vi "example_tinygo_sht31_monitor.vi"() -> ()   [LabVIEW 2020]
uses:
  <vilib>/Instr/_visa.llb/VISA Configure Serial Port (Instr).vi
  <vilib>/ptbypt/NI_PtbyPt.lvlib
panel:
  out "TimeStamp":timestamp
  out "dT (ms)":u32
  out "Error Count":u32
  out "Waveform Chart":cluster{dbl, dbl}(graph)
  in  "Brn Clear":bool
  in  "Btn Send":bool
  in  "cmd string":string
  out "rcvdata counter":i32
  out "rcvdata string":string
  in  "que type":cluster{"event":string, "param":variant}
  out "read buffer":string
  in  "Btn stop":bool
  in  "VISA resource name":refnum<visa-resource-name>
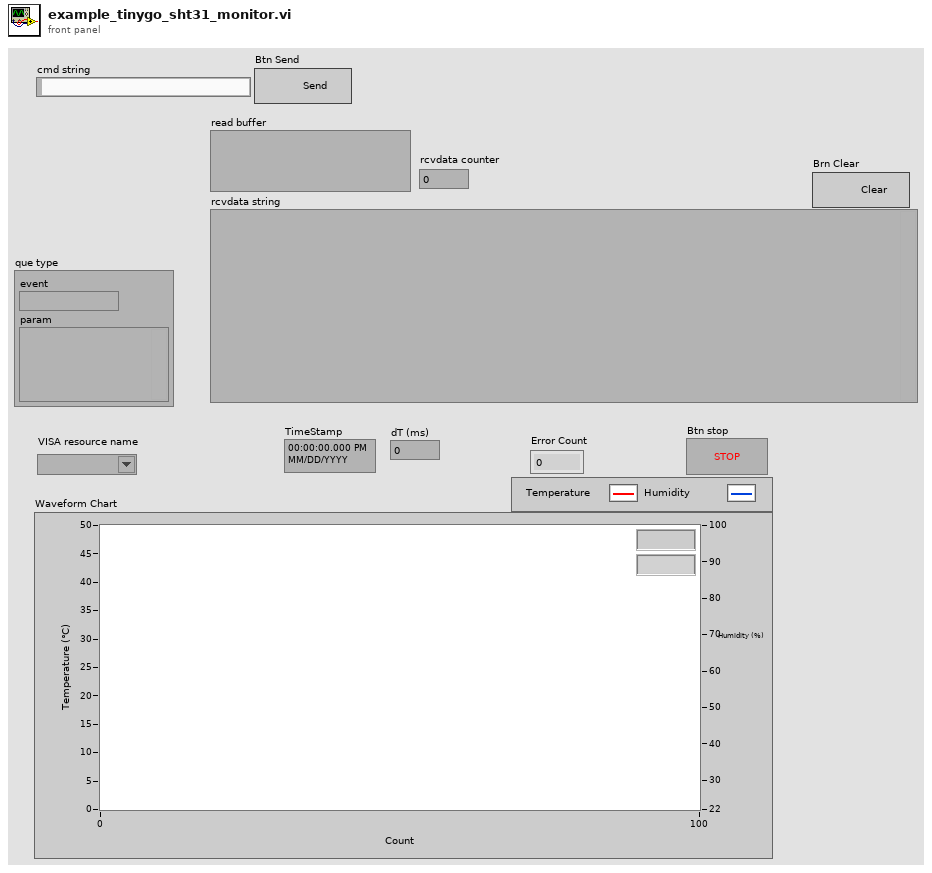
[diagram p1: front panel]
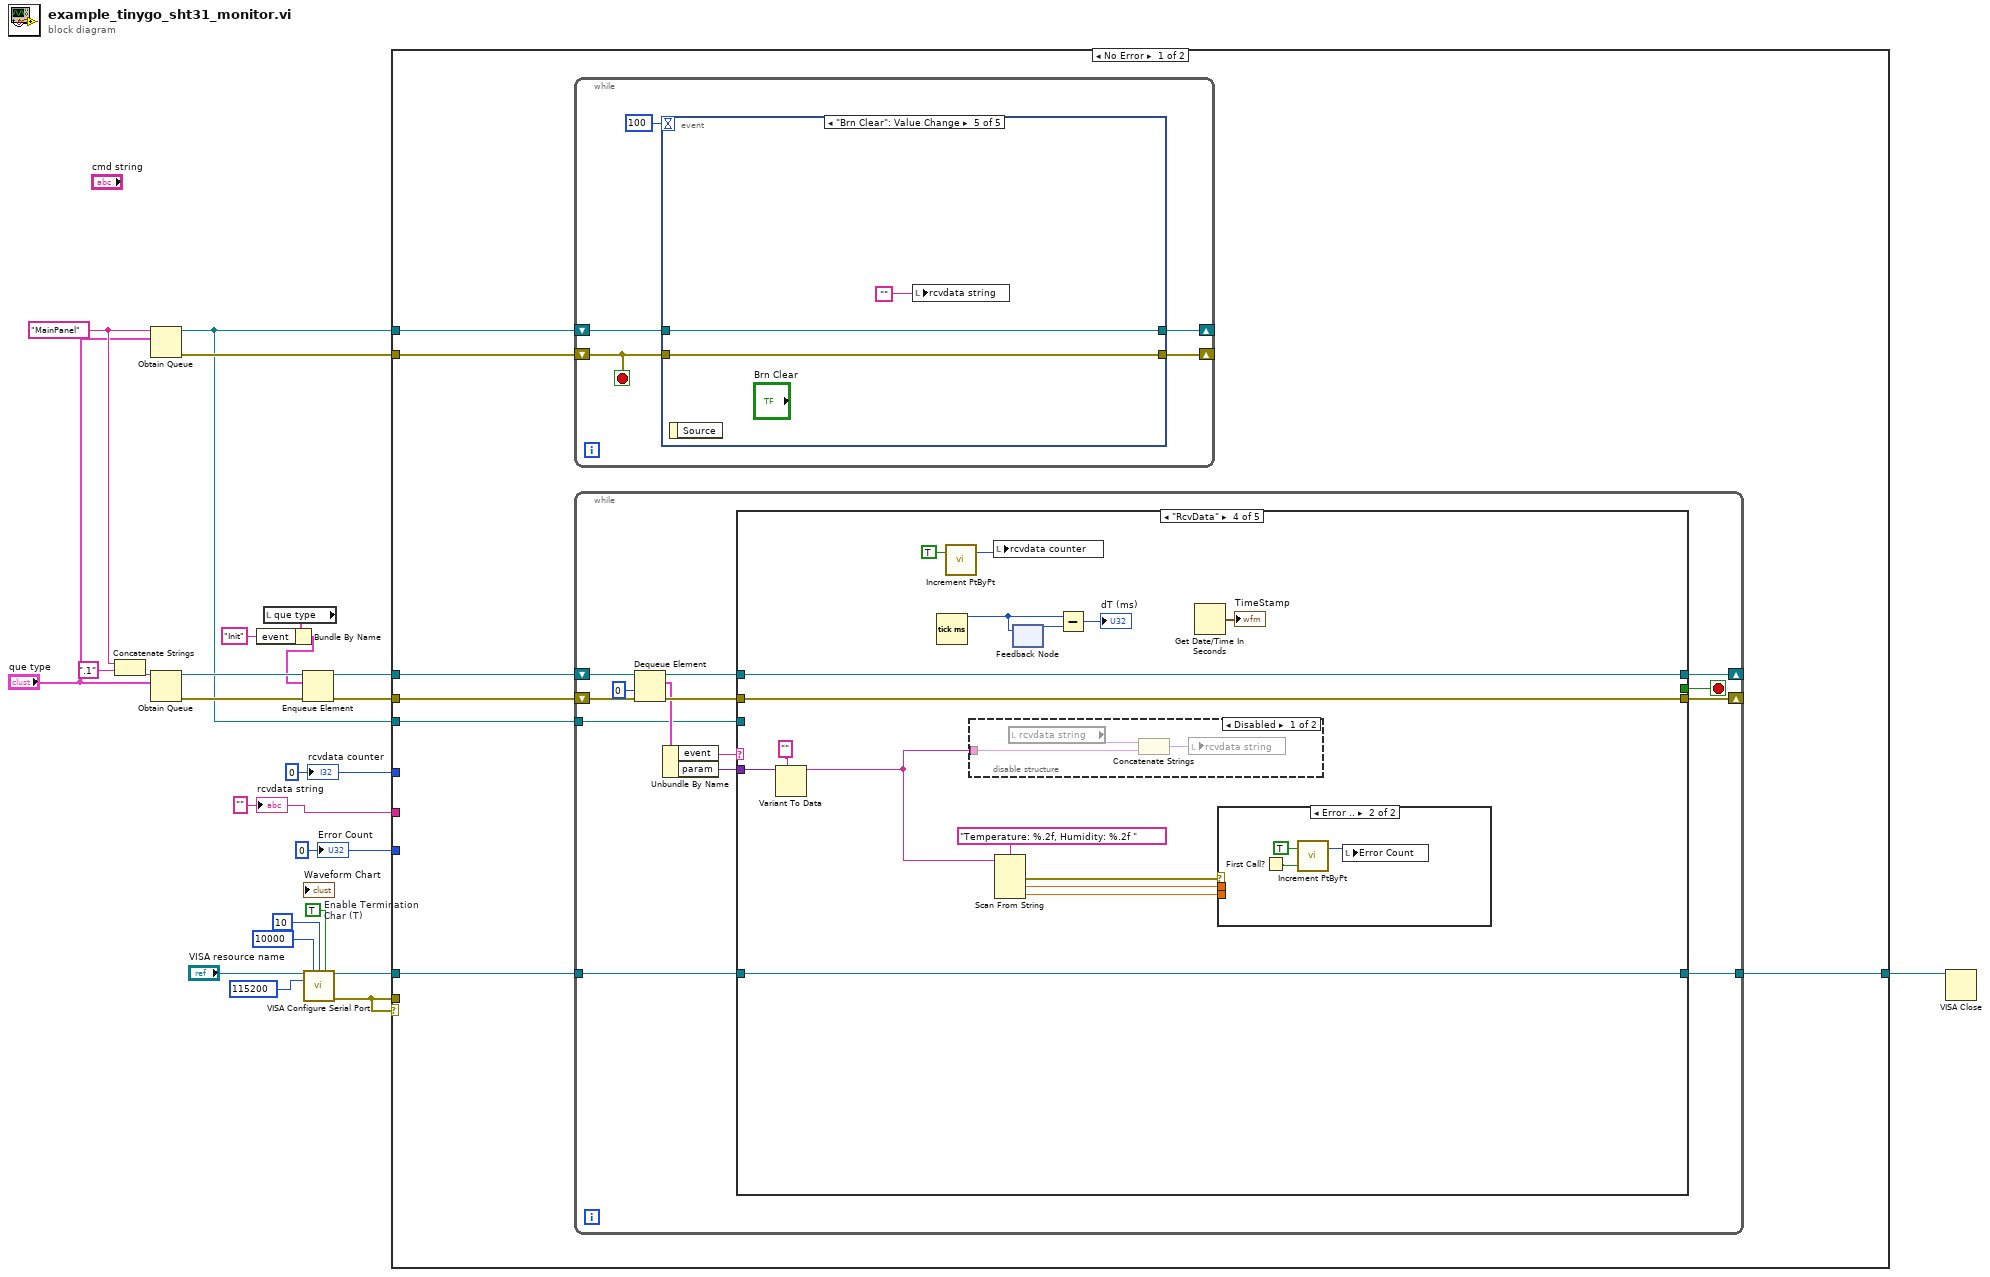
[diagram p0: block diagram]
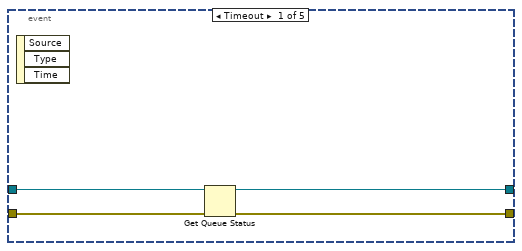
[diagram p2: hidden frame]
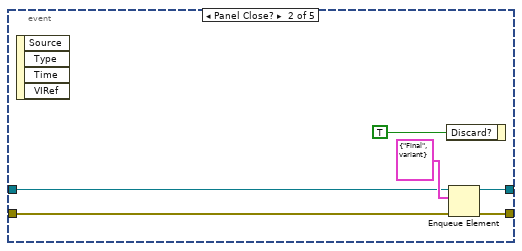
[diagram p3: hidden frame]
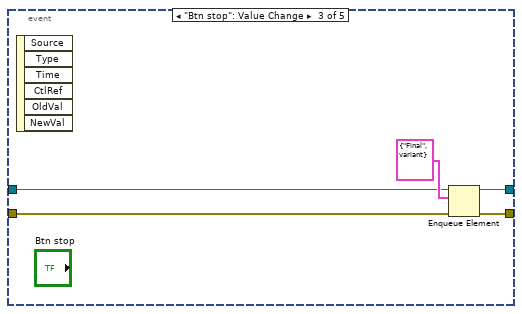
[diagram p4: hidden frame]
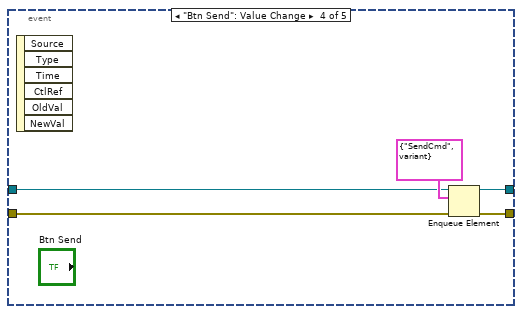
[diagram p5: hidden frame]
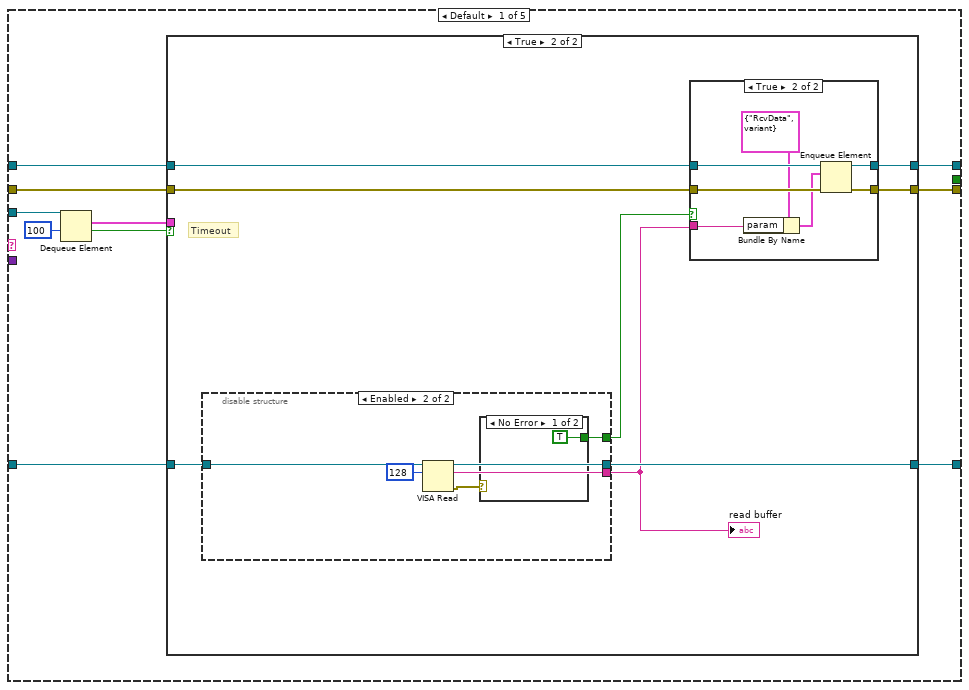
[diagram p6: hidden frame]
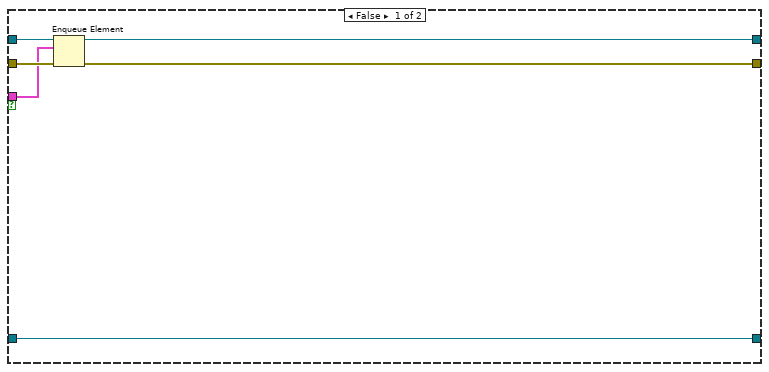
[diagram p7: hidden frame]
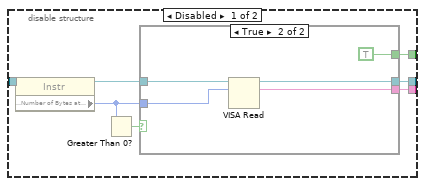
[diagram p8: hidden frame]
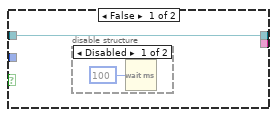
[diagram p9: hidden frame]
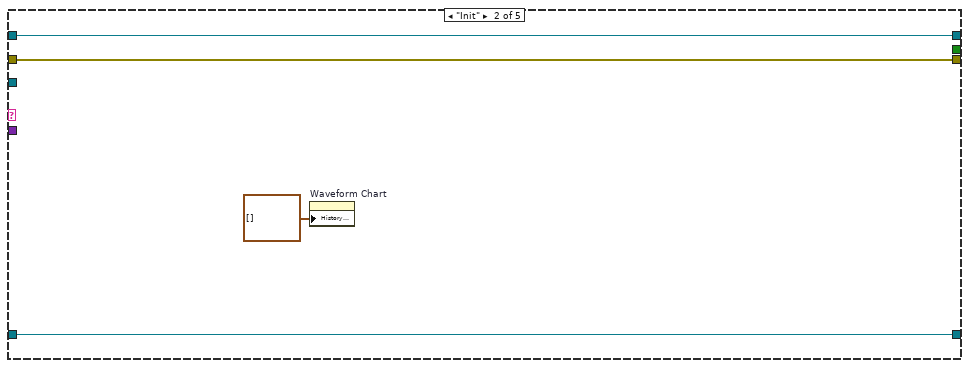
[diagram p13: hidden frame]
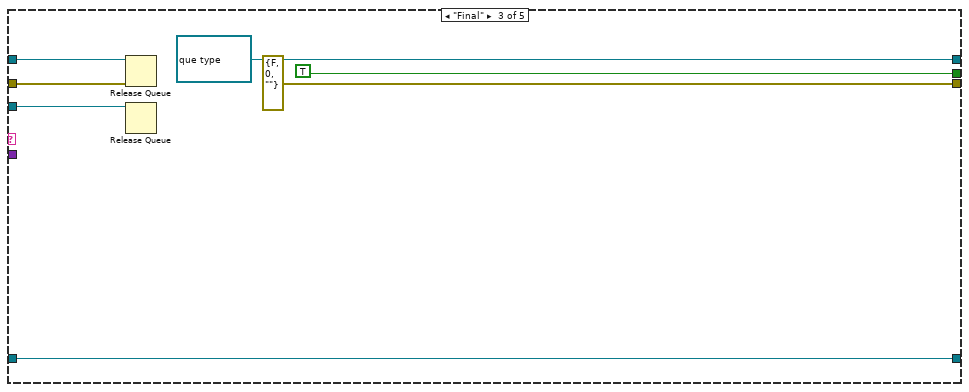
[diagram p14: hidden frame]
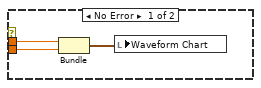
[diagram p15: hidden frame]
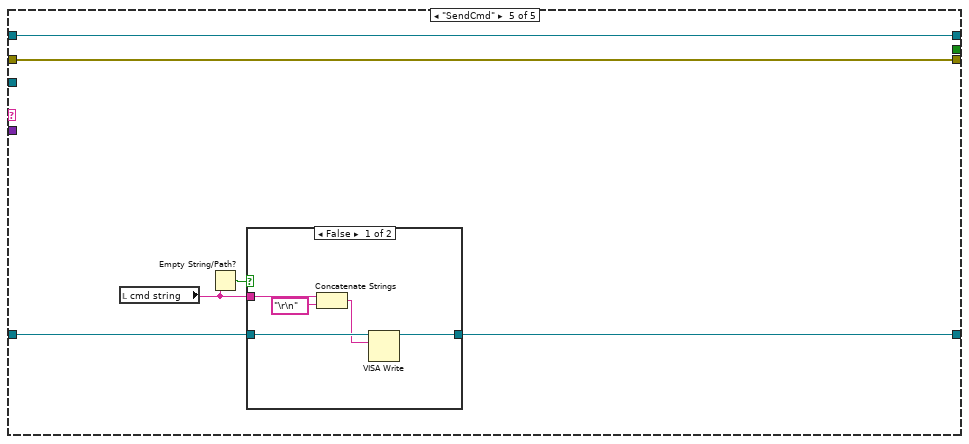
[diagram p17: hidden frame]
diagram:
  w1 = u32 0 ("Error Count")
  w2 = "" ("cmd string")
  w3 = 0 ("rcvcmd counter")
  w8 = "MainPanel" ("name (unnamed)")
  w19 = TRUE  # Enable Termination Char (T)
  n1 = Concatenate Strings(w8, ".1" ("string")) -> (w7:string)
  n2 = Obtain Queue(name (unnamed)=w8, element data type="que type") -> (queue out=w5:refnum<queue>, error out=w9:errorcluster)  [unwired: 3 in, 1 out]
  n3 = Obtain Queue(name (unnamed)=w7, element data type="que type") -> (queue out=w16:refnum<queue>, error out=w10:errorcluster)  [unwired: 3 in, 1 out]
  n4 = local read "que type"() -> (w14:cluster{"event":string, "param":variant})
  n5 = Bundle By Name(cluster=w14, "event"="Init") -> (w12:cluster{"event":string, "param":variant})
  n6 = Enqueue Element(queue=w16, element=w12, error in (no error)=w10) -> (queue out=w15:refnum<queue>, error out=w11:errorcluster)  [unwired: 1 in, 1 out]
  n7 = call-poly "VISA Configure Serial Port"("VISA resource name"="VISA resource name", "timeout (10sec)"=u32 10000, "termination char\n(0xA = '\\n' = LF)"=u8 10 ("termination char\n(0xA = '\\n' = LF)"), "Enable Termination\nChar (T)"=w19, "baud rate (9600)"=u32 115200) -> ("VISA resource name out"=w22:refnum<visa-resource-name>, "error out"=w23:errorcluster)  [unwired: 9 in]
  n8 = case shown="No Error" w23 {
    tunnel: w23 -> [_ _]
    tunnel: w22 -> [w31 w175]
    tunnel: [w30 w175] -> w18
    tunnel: w15 -> [w29 _]
    tunnel: w11 -> [w28 _]
    tunnel: w5 -> [w27 _]
    tunnel: w9 -> [w26 _]
    tunnel: w5 -> [w25 _]
    tunnel: w3 -> [_ _]
    tunnel: w2 -> [_ _]
    tunnel: w1 -> [_ _]
    frame No Error {
      n9 = while {
        shift-right: [w32] -> _
        shift-left: w26 -> [w35]
        shift-right: [w33] -> _
        shift-left: w27 -> [w34]
        stop <- w35 stop-if-true
        n10 = event shown="[4] \"Brn Clear\": Value Change" {
          selector: _ -> [_ _ _ _ _]
          dyn-events: _ -> [_ _ _ _ _]
          timeout: 100 -> [_ _ _ _ _]
          tunnel: w35 -> [w39 w41 w47 w52 w58]
          tunnel: w34 -> [w40 w42 w48 w53 w59]
          tunnel: [w38 w43 w49 w54 w59] -> w33
          tunnel: [w37 w44 w50 w55 w58] -> w32
          event Timeout {
            n11 = event-data() -> ()  [unwired: 1 in, 3 out]
            n12 = Get Queue Status(queue=w40, error in (no error)=w39) -> (queue out=w38:refnum<queue>, error out=w37:errorcluster)  [unwired: 1 in, 6 out]
          }
          event Panel Close? {
            n13 = event-data() -> ()  [unwired: 1 in, 4 out]
            n14 = event-data("Discard?"=TRUE) -> ()  [unwired: 1 in, 1 out]
            n15 = Enqueue Element(queue=w42, element=cluster{"event":string, "param":variant} {"event"="Final", "param"=variant}, error in (no error)=w41) -> (queue out=w43:refnum<queue>, error out=w44:errorcluster)  [unwired: 1 in, 1 out]
          }
          event "Btn stop": Value Change {
            n16 = event-data() -> ()  [unwired: 1 in, 6 out]
            n17 = Enqueue Element(queue=w48, element=cluster{"event":string, "param":variant} {"event"="Final", "param"=variant}, error in (no error)=w47) -> (queue out=w49:refnum<queue>, error out=w50:errorcluster)  [unwired: 1 in, 1 out]
          }
          event "Btn Send": Value Change {
            n18 = event-data() -> ()  [unwired: 1 in, 6 out]
            n19 = Enqueue Element(queue=w53, element=cluster{"event":string, "param":variant} {"event"="SendCmd", "param"=variant}, error in (no error)=w52) -> (queue out=w54:refnum<queue>, error out=w55:errorcluster)  [unwired: 1 in, 1 out]
          }
          event "Brn Clear": Value Change {
            n20 = event-data() -> ()  [unwired: 1 in, 1 out]
            n21 = local write "rcvdata string"("") -> ()
          }
        }
      }
      n22 = while {
        tunnel: w31 -> [w72]
        tunnel: [w73] -> w30
        shift-right: [w62] -> _
        shift-left: w29 -> [w71]
        shift-right: [w61] -> _
        shift-left: w28 -> [w69]
        tunnel: w25 -> [w63]
        stop <- w60 stop-if-true
        n23 = Dequeue Element(queue=w71, timeout in ms (-1)=0, error in (no error)=w69) -> (queue out=w70:refnum<queue>, element=w66:cluster{"event":string, "param":variant}, error out=w68:errorcluster)  [unwired: 1 out]
        n24 = Unbundle By Name(w66) -> ("event"=w65:string, "param"=w64:variant)
        n25 = case shown="\"RcvData\"" w65 {
          tunnel: [w83 w128 w137 w151 w165] -> w73
          tunnel: w72 -> [w82 w128 w137 w151 w166]
          tunnel: w70 -> [w78 w130 w136 w153 w168]
          tunnel: w68 -> [w76 w129 w135 w152 w167]
          tunnel: w64 -> [_ _ _ w150 _]
          tunnel: w63 -> [w81 _ w134 _ _]
          tunnel: [w77 w130 refnum<queue> refnum ("queue out") w153 w168] -> w62
          tunnel: [w75 w129 errorcluster {"status"=FALSE, "code"=0, "source"=""} ("error out") w152 w167] -> w61
          tunnel: [_ _ TRUE _ _] -> w60
          frame Default {
            n26 = Dequeue Element(queue=w81, timeout in ms (-1)=100) -> (element=w74:cluster{"event":string, "param":variant}, timed out?=w79:bool)  [unwired: 1 in, 2 out]
            n27 = case shown="True" w79 {
              tunnel: [w84 w95] -> w83
              tunnel: w82 -> [w84 w96]
              tunnel: w78 -> [w88 w91]
              tunnel: [w86 w94] -> w77
              tunnel: [w87 w93] -> w75
              tunnel: w76 -> [w87 w92]
              tunnel: w74 -> [w85 _]
              frame False {
                n28 = Enqueue Element(queue=w88, element=w85) -> (queue out=w86:refnum<queue>)  [unwired: 2 in, 2 out]
              }
              frame True {
                # "Timeout"
                n29 = disable-structure shown="Enabled" {
                  disable-tunnel: w96 -> [w100 w113]
                  disable-tunnel: [w99 w116] -> w95
                  disable-tunnel: [w98 w115] -> w89
                  disable-tunnel: [w97 w114] -> w90
                  frame Disabled {
                    n30 = property class="Instr"(reference=w100) -> (reference out=w103:refnum<visa-resource-name>, "Serial Settings:Number of Bytes at Serial Port"=w102:u32)  [unwired: 1 in, 1 out]
                    n31 = Greater Than 0?(x=w102) -> (x > 0?=w101:bool)
                    n32 = case shown="True" w101 {
                      tunnel: [w104 w110] -> w99
                      tunnel: w103 -> [w104 w109]
                      tunnel: w102 -> [_ w108]
                      tunnel: [_ w107] -> w98
                      tunnel: [_ TRUE] -> w97
                      frame False {
                        n33 = disable-structure shown="Disabled" {
                          frame Disabled {
                            n34 = Wait (ms)(milliseconds to wait=u32 100) -> ()  [unwired: 1 out]
                          }
                          frame Enabled {
                          }
                        }
                      }
                      frame True {
                        n35 = VISA Read(VISA resource name=w109, byte count=w108) -> (VISA resource name out=w110:refnum<visa-resource-name>, read buffer=w107:string)  [unwired: 1 in, 2 out]
                      }
                    }
                  }
                  frame Enabled {
                    n36 = VISA Read(VISA resource name=w113, byte count=u32 128) -> (VISA resource name out=w116:refnum<visa-resource-name>, read buffer=w115:string, error out=w111:errorcluster)  [unwired: 1 in, 1 out]
                    n37 = case shown="No Error" w111 {
                      tunnel: [TRUE _] -> w114
                      frame No Error {
                      }
                      frame Error {
                      }
                    }
                  }
                }
                "read buffer" <- w89
                n38 = case shown="True" w90 {
                  tunnel: [w119 w126] -> w94
                  tunnel: [w118 w125] -> w93
                  tunnel: w92 -> [w118 w124]
                  tunnel: w91 -> [w119 w123]
                  tunnel: w89 -> [_ w120]
                  frame False {
                  }
                  frame True {
                    n39 = Bundle By Name(cluster=cluster{"event":string, "param":variant} {"event"="RcvData", "param"=variant}, "param"=w120) -> (w121:cluster{"event":string, "param":variant})
                    n40 = Enqueue Element(queue=w123, element=w121, error in (no error)=w124) -> (queue out=w126:refnum<queue>, error out=w125:errorcluster)  [unwired: 1 in, 1 out]
                  }
                }
              }
            }
          }
          frame "Init" {
            n41 = property on="Waveform Chart" class="WFChart (strict)"("History Data"=cluster{dbl, dbl}[] []) -> ()  [unwired: 2 in, 2 out]
          }
          frame "Final" {
            n42 = Release Queue(queue=w136, error in (no error)=w135) -> ()  [unwired: 1 in, 3 out]
            n43 = Release Queue(queue=w134) -> ()  [unwired: 2 in, 3 out]
          }
          frame "RcvData" {
            n44 = Variant To Data(type="", Variant=w150) -> (data=w145:string)  [unwired: 1 in, 1 out]
            n45 = Tick Count (ms)() -> (millisecond timer value=w140:u32)
            n46 = call <vilib>:"Increment PtByPt.vi"("activate"=TRUE) -> ("counter"=w148:u32)  [unwired: 1 in, 1 out]
            n47 = disable-structure shown="Disabled" {
              disable-tunnel: w145 -> [w160 _]
              frame Disabled {
                n48 = local read "rcvdata string"() -> (w162:string)
                n49 = Concatenate Strings(w162, w160) -> (w161:string)
                n50 = local write "rcvdata string"(w161) -> ()
              }
              frame Enabled {
              }
            }
            n51 = local write "rcvdata counter"(w148) -> ()
            n52 = Scan From String(format string="Temperature: %.2f, Humidity: %.2f ", input string=w145) -> (error out=w142:errorcluster, output 1=w144:dbl, output 2=w143:dbl)  [unwired: 4 in, 2 out]
            n53 = feedback-in #1(w140) -> ()
            n54 = feedback #1() -> (w141:u32)  [unwired: 1 in]
            n55 = Subtract(x=w140, y=w141) -> (x-y=→"dT (ms)":u32)
            n56 = Get Date/Time In Seconds() -> (seconds since 1Jan1904=→"TimeStamp":timestamp)
            n57 = case shown="Error .." w142 {
              tunnel: w144 -> [w156 _]
              tunnel: w143 -> [w155 _]
              frame No Error {
                n58 = Bundle(w156, w155) -> (w154:cluster{dbl, dbl})  [unwired: 1 in]
                n59 = local write "Waveform Chart"(w154) -> ()
              }
              frame Error {
                n60 = First Call?() -> (First Call?: T/F=w159:bool)
                n61 = call <vilib>:"Increment PtByPt.vi"("initialize"=w159, "activate"=TRUE) -> ("counter"=w157:u32)  [unwired: 1 out]
                n62 = local write "Error Count"(w157) -> ()
              }
            }
          }
          frame "SendCmd" {
            n63 = local read "cmd string"() -> (w163:string)
            n64 = Empty String/Path?(string/path=w163) -> (empty?=w164:bool)
            n65 = case shown="False" w164 {
              tunnel: w166 -> [w173 w174]
              tunnel: [w172 w174] -> w165
              tunnel: w163 -> [w171 _]
              frame False {
                n66 = Concatenate Strings(w171, "\r\n") -> (w170:string)
                n67 = VISA Write(VISA resource name=w173, write buffer=w170) -> (VISA resource name out=w172:refnum<visa-resource-name>)  [unwired: 1 in, 2 out]
              }
              frame True {
              }
            }
          }
        }
      }
    }
    frame Error {
    }
  }
  n68 = VISA Close(VISA resource name=w18) -> ()  [unwired: 1 in, 1 out]
  "rcvdata counter" <- w3
  "rcvdata string" <- w2
  "Error Count" <- w1
